vi "Result.Remove Heading Info from UUT Result Attributes.vi"(9 "Remove Heading Values":bool=TRUE, 10 "Remove Headings":bool, 11 "Data":T1={"#attributes"={"Version"="MTE_1.0.0"}, "Station"={"Name"="", "PN"="", "SN"="", "Rev"="", "PC Name"="", "Location"="", "HW_Config"={"HW_Item"=[]}, "SW_Config"={"SW_Item"=[]}}, "Test Run"={"Operator"="", "Start Time"=timestamp(0 s since 1904-01-01), "Duration(s)"=0.0, "Mode"="", "Comment"="", "ProcessStep"=""}, "Test Sequence"={"Name"="", "Config"={"Config_Item"=[]}}, "UUTs"={"UUT"=[]}} {"UUTs"."UUT"."Measurements"."Measurement"."Status" items=["LOG", "PASS", "FAIL", "ERROR"]}) -> (3 "Data Out":T1={"#attributes"={"Version"="MTE_1.0.0"}, "Station"={"Name"="", "PN"="", "SN"="", "Rev"="", "PC Name"="", "Location"="", "HW_Config"={"HW_Item"=[]}, "SW_Config"={"SW_Item"=[]}}, "Test Run"={"Operator"="", "Start Time"=timestamp(0 s since 1904-01-01), "Duration(s)"=0.0, "Mode"="", "Comment"="", "ProcessStep"=""}, "Test Sequence"={"Name"="", "Config"={"Config_Item"=[]}}, "UUTs"={"UUT"=[]}} {"UUTs"."UUT"."Measurements"."Measurement"."Status" items=["LOG", "PASS", "FAIL", "ERROR"]})   [LabVIEW 2018]
uses:
  Result XML/TestResult.FullResultData.ctl
  Result XML/TestResult.Station Info.ctl
  Result XML/TestResult.HW Item.ctl
  Result XML/TestResult.SW Item.ctl
  Result XML/TestResult.Test Run Info.ctl
  Result XML/TestResult.Test Info.ctl
  Result XML/TestResult.UUT Result.ctl
  Result XML/TestResult.Symptom.ctl
  Result XML/TestResult.Symptom.State.ctl
  Result.Measurement Item.ctl
  Result.Measurement and Attribute Item Status.ctl
  Result XML/TestResult.UUTInfo.ctl
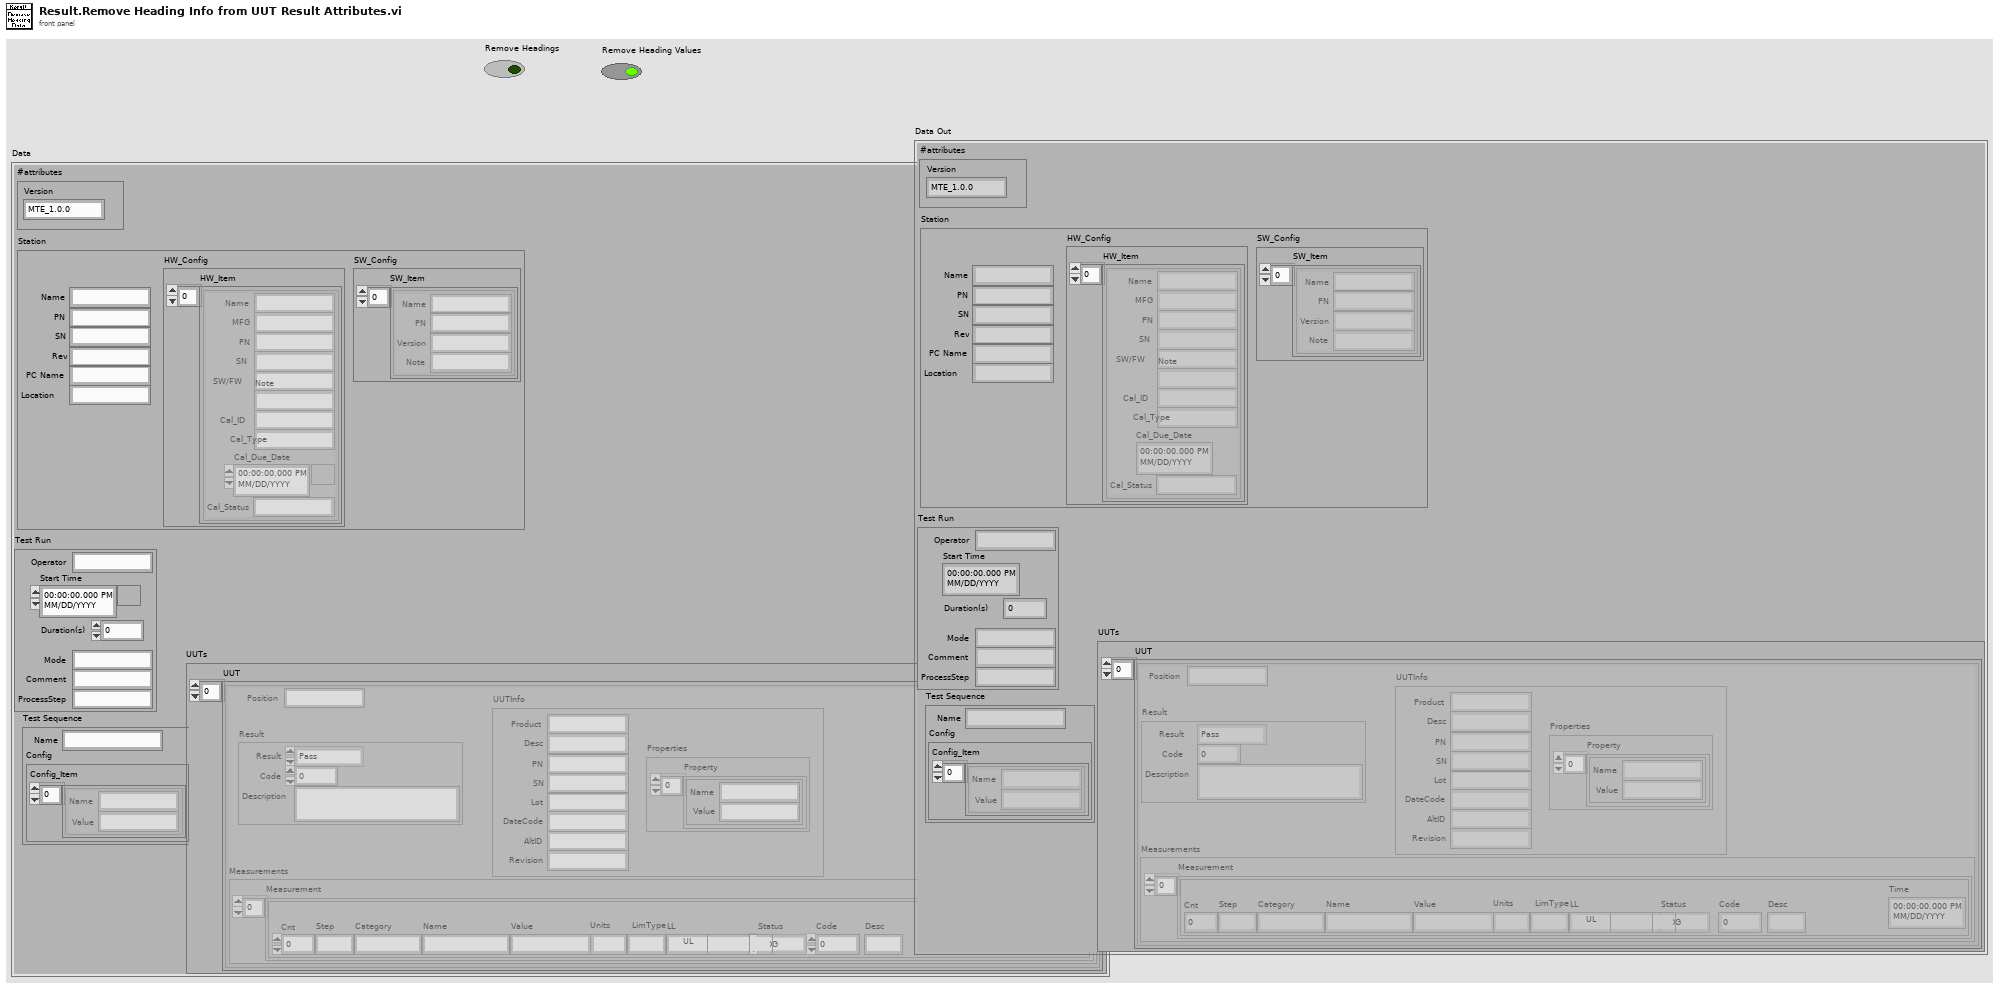
[diagram p1: front panel]
types:
  T1 = typedef "TestResult.FullResultData.ctl" = cluster{"#attributes":cluster{"Version":string}, "Station":T2, "Test Run":T5, "Test Sequence":T6, "UUTs":cluster{"UUT":T7[]}}
  T2 = typedef "TestResult.Station Info.ctl" = cluster{"Name":string, "PN":string, "SN":string, "Rev":string, "PC Name":string, "Location":string, "HW_Config":cluster{"HW_Item":T3[]}, "SW_Config":cluster{"SW_Item":T4[]}}
  T3 = typedef "TestResult.HW Item.ctl" = cluster{"Name":string, "MFG":string, "PN":string, "SN":string, "SW/FW":string, "Note":string, "Cal_ID":string, "Cal_Type":string, "Cal_Due_Date":timestamp, "Cal_Status":string}
  T4 = typedef "TestResult.SW Item.ctl" = cluster{"Name":string, "PN":string, "Version":string, "Note":string}
  T5 = typedef "TestResult.Test Run Info.ctl" = cluster{"Operator":string, "Start Time":timestamp, "Duration(s)":dbl, "Mode":string, "Comment":string, "ProcessStep":string}
  T6 = typedef "TestResult.Test Info.ctl" = cluster{"Name":string, "Config":cluster{"Config_Item":cluster{"Name":string, "Value":string}[]}}
  T7 = typedef "TestResult.UUT Result.ctl" = cluster{"Position":string, "Result":T8, "Measurements":cluster{"Measurement":T10[]}, "UUTInfo":T12}
  T8 = typedef "TestResult.Symptom.ctl" = cluster{"Result":T9, "Code":i32, "Description":string}
  T9 = typedef "TestResult.Symptom.State.ctl" = enum16{"Pass", "Fail", "Error", "Aborted", "Completed", "Logged"}
  T10 = typedef "Result.Measurement Item.ctl" = cluster{"Cnt":i32, "Step":string, "Category":string, "Name":string, "Value":string, "Units":string, "LimType":string, "LL":string, "UL":string, "Status":T11, "Code":i32, "Desc":string, "Time":timestamp}
  T11 = typedef "Result.Measurement and Attribute Item Status.ctl" = i32
  T12 = typedef "TestResult.UUTInfo.ctl" = cluster{"Product":string, "Desc":string, "PN":string, "SN":string, "Lot":string, "DateCode":string, "AltID":string, "Revision":string, "Properties":cluster{"Property":cluster{"Name":string, "Value":string}[]}}
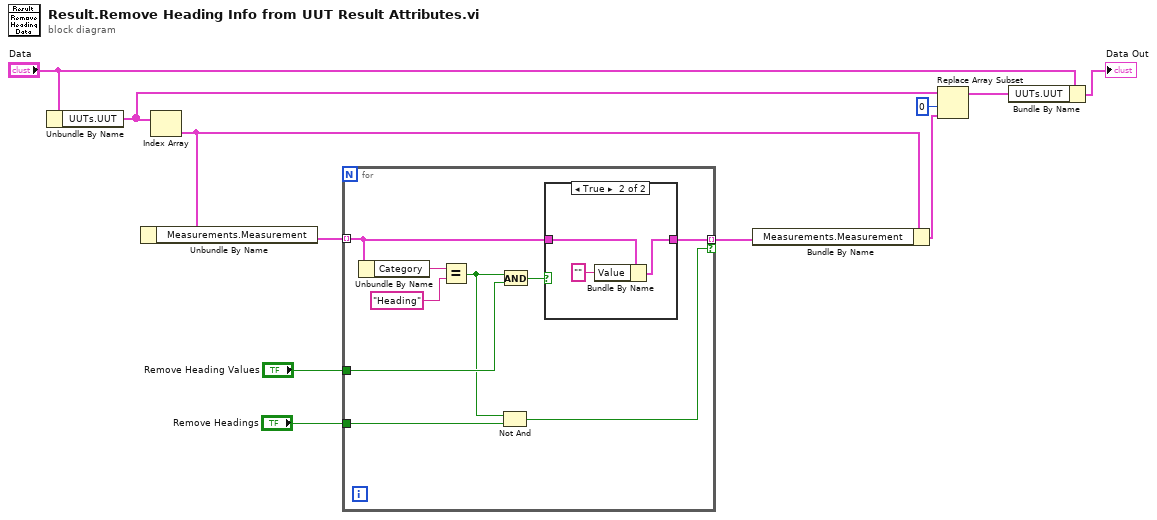
[diagram p0: block diagram]
diagram:
  n1 = Unbundle By Name("Data") -> ("UUTs.UUT"=w10:T7[])
  n2 = Index Array(array=w10) -> (element=w6:T7)  [unwired: 1 in]
  n3 = Unbundle By Name(w6) -> ("Measurements.Measurement"=w9:T10[])
  n4 = for {
    tunnel: w9 -> [w18] mode=indexing
    tunnel: [w17] -> w7 mode=indexing if=w12
    tunnel: "Remove Heading Values" -> [w15]
    tunnel: "Remove Headings" -> [w13]
    n5 = Unbundle By Name(w18) -> ("Category"=w20:string)
    n6 = Equal?(x=w20, y="Heading") -> (x = y?=w14:bool)
    n7 = Not And(1:w13, 2:w14) -> (0:w12:bool)
    n8 = And(x=w14, y=w15) -> (x .and. y?=w16:bool)
    n9 = case shown="True" w16 {
      tunnel: w18 -> [w21 w24]
      tunnel: [w21 w22] -> w17
      frame False {
      }
      frame True {
        n10 = Bundle By Name(cluster=w24, "Value"="") -> (w22:T10)
      }
    }
  }
  n11 = Bundle By Name(cluster=w6, "Measurements.Measurement"=w7) -> (w8:T7)
  n12 = Replace Array Subset(array=w10, new element=w8, index=0) -> (w4:T7[])
  n13 = Bundle By Name(cluster="Data", "UUTs.UUT"=w4) -> (→"Data Out":T1)
